vi "Comments.Create Lockin Sampling Description.vi"(7 "error in (no error)":errorcluster, 10 "Control Experiment":refnum<class "Control Experiment.lvclass">) -> (0 "error out":errorcluster, 2 "Sampling Section":string, 3 "Control Experiment out":refnum<class "Control Experiment.lvclass">)   [LabVIEW 2019, in "Control Experiment.lvclass"]
uses:
  Control Experiment.lvclass
  Control Experiment.lvclass/Control Experiment.ctl
  <userlib>/LevyLab/Instrument Framework/Instrument Types/Lockin/Instrument.LockinAPI.lvclass
  <userlib>/LevyLab/PLYM/YAML.lvclass
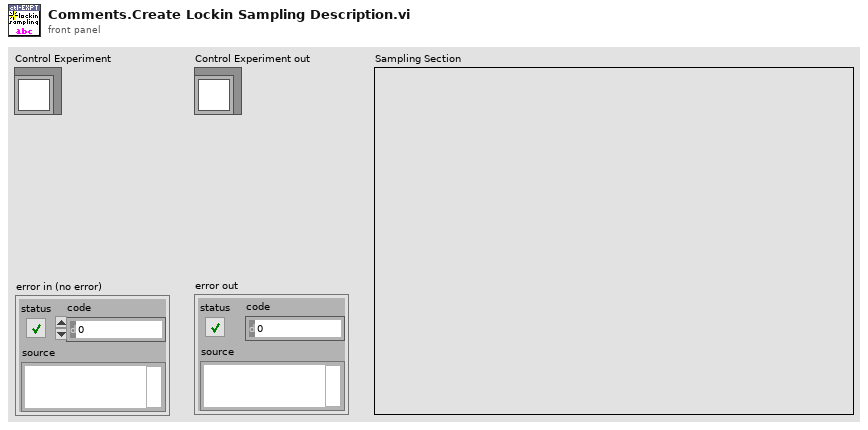
[diagram p1: front panel]
types:
  T1 = typedef "Instrument.LockinAPI.lvclass/LockinAPI.Sampling.Sampling--Cluster.ctl" = cluster{"Fs":dbl, "#s":i32}
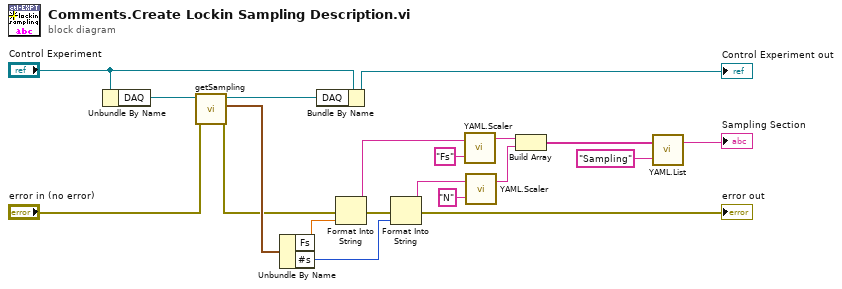
[diagram p0: block diagram]
diagram:
  n1 = Unbundle By Name("Control Experiment") -> ("DAQ"=w3:refnum<class "Instrument.LockinAPI.lvclass">)
  n2 = call-dynamic "getSampling.vi"("error in (no error)"="error in (no error)", "Instrument.LockinAPI in"=w3) -> ("error out"=w2:errorcluster, "sampling"=w6:T1, "Instrument.LockinAPI out"=w4:refnum<class "Instrument.LockinAPI.lvclass">)  [unwired: 7 in]
  n3 = Unbundle By Name(w6) -> ("Fs"=w19:dbl, "#s"=w8:i32)
  n4 = Bundle By Name(cluster="Control Experiment", "DAQ"=w4) -> (→"Control Experiment out":refnum<class "Control Experiment.lvclass">)
  n5 = Format Into String(error in=w2, w19) -> (resulting string=w14:string, error out=w20:errorcluster)  [unwired: 2 in]
  n6 = Format Into String(error in=w20, w8) -> (resulting string=w16:string, error out=→"error out":errorcluster)  [unwired: 2 in]
  n7 = call <userlib>:"YAML.Scaler.vi"("Key"="Fs", "Scaler"=w14) -> ("Output"=w11:string)  [unwired: 1 in]
  n8 = call <userlib>:"YAML.Scaler.vi"("Key"="N", "Scaler"=w16) -> ("Output"=w10:string)  [unwired: 1 in]
  n9 = Build Array(w11, w10) -> (w9:string[])
  n10 = call <userlib>:"YAML.List.vi"("Key"="Sampling" ("string"), "lines"=w9) -> ("Output"=→"Sampling Section":string)  [unwired: 1 in]
